vi "FPGA Test Shell.vi"() -> ()   [LabVIEW 2014]
uses:
  <vilib>/FPGAPlugInAG/sbRIO-9636/niLvFpga_Open_sbRIO-9636.vi
  <vilib>/rvi/interface/common/dynamic/niFpgaDynamicAddResources.vi
  <vilib>/FPGAPlugInAG/Dynamic/niLvFpga_Reset_Dynamic.vi
  <vilib>/FPGAPlugInAG/Dynamic/niLvFpga_Run_Dynamic.vi
  <vilib>/Utility/error.llb/Error Cluster From Error Code.vi
  <vilib>/rvi/errors/niLvFpgaAdjustHostInterfaceError.vi
  <vilib>/FPGAPlugInAG/Dynamic/niLvFpga_Close_Dynamic.vi
  <vilib>/rvi/interface/nirviOpenFPGA/nirviOpenFPGA.xnode
  FPGA Bitfiles/Exercise2-FPGASo_FPGATarget_Exercise2Solutio_5A33415C.lvbitx
  <vilib>/rvi/interface/nirviMethod/nirviMethod.xnode
  <vilib>/rvi/interface/nirviReadWriteControl/nirviReadWriteControl.xnode
  <vilib>/rvi/interface/nirviCloseFPGA/nirviCloseFPGA.xnode
  NiFpgaLv.dll
  <vilib>/rvi/interface/Simulation/niFpgaSimulationCallBeginRW.vi
panel:
  out "FPGA Display Command":T1(ring)
  in  "stop":bool
  out "Battery State":enum16{"Charged", "Running", "Low Batt"}(ring)
  out "Temp Warning":bool
  out "Temp":fxp<+/-,32,13> format="%#_3g"
  out "Voltage":fxp<+/-,24,5> format="%#_3g"
  out "RPM":fxp<+,32,16> format="%#_3g"
  in  "Max Temp":fxp<+/-,32,13>=25.0
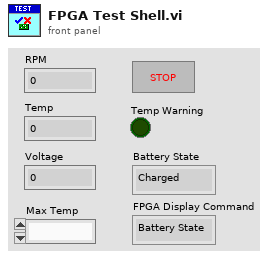
[diagram p1: front panel]
types:
  T1 = enum16{"Battery State", "RPM", "Temp", "Voltage"}
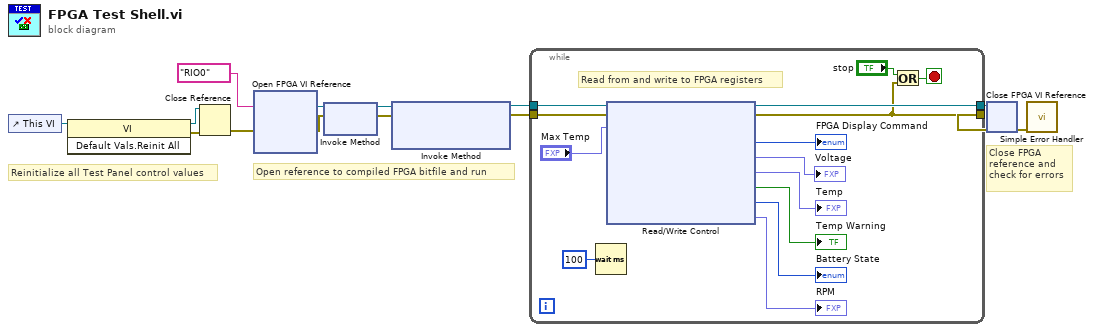
[diagram p0: block diagram]
diagram:
  # "Close FPGA \nreference and\ncheck for errors"
  # "Open reference to compiled FPGA bitfile and run"
  # "Reinitialize all Test Panel control values"
  n1 = control-ref of="This VI"() -> (w4:refnum<vi>)
  n2 = invoke class="VI" method="Default Vals.Reinit All"(reference=w4) -> (reference out=w1:refnum<vi>, error out=w3:errorcluster)  [unwired: 2 in, 1 out]
  n3 = Close Reference(reference=w1, error in (no error)=w3) -> (error out=w2:errorcluster)
  n4 = xnode "Open FPGA VI Reference"("error in"=w2, "resource name"=tag "RIO0") -> ("FPGA VI Reference Out"=w13:refnum<k20>, "error out"=w9:errorcluster)
  n5 = xnode "Invoke Method"("FPGA VI Reference In"=w13, "error in"=w9) -> ("FPGA VI Reference Out"=w12:refnum<k20>, "error out"=w8:errorcluster)
  n6 = xnode "Invoke Method"("FPGA VI Reference In"=w12, "error in"=w8) -> ("FPGA VI Reference Out"=w11:refnum<k20>, "error out"=w7:errorcluster)  [unwired: 1 in]
  n7 = while {
    tunnel: w11 -> [w28]
    tunnel: [w21] -> w10
    tunnel: w7 -> [w20]
    tunnel: [w17] -> w6
    stop <- w19 stop-if-true
    # "Read from and write to FPGA registers"
    n8 = Wait (ms)(milliseconds to wait=u32 100) -> ()  [unwired: 1 out]
    n9 = xnode "Read/Write Control"("FPGA VI Reference In"=w28, "error in"=w20, "Max Temp"="Max Temp") -> ("FPGA VI Reference Out"=w21:refnum<k20>, "error out"=w17:errorcluster, "FPGA Display Command"=→"FPGA Display Command":T1, "Voltage"=→"Voltage":fxp<+/-,24,5>, "Temp"=→"Temp":fxp<+/-,32,13>, "Temp Warning"=→"Temp Warning":bool, "Battery State"=→"Battery State":enum16{"Charged", "Running", "Low Batt"}, "RPM"=→"RPM":fxp<+,32,16>)
    n10 = Or(x="stop", y=w17) -> (x .or. y?=w19:bool)
  }
  n11 = xnode "Close FPGA VI Reference"("FPGA VI Reference In"=w10, "error in"=w6) -> ("error out"=w5:errorcluster)
  n12 = call <vilib>:"Simple Error Handler.vi"("error in (no error)"=w5) -> ()  [unwired: 4 in, 5 out]
